vi "NK11003_ONOFF.vi"(8 "error in":errorcluster caption="错误输入（无错误）", 10 "启停":enum16{"启动", "停止"}(ring), 11 "MyIndex":u8) -> (0 "error out":errorcluster caption="错误输出", 3 "OK?":bool)   [LabVIEW 2015]
uses:
  <vilib>/Instr/_visa.llb/VISA Configure Serial Port (Instr).vi
panel:
  out "VISA":refnum<visa-resource-name> caption="VISA资源名称输出"
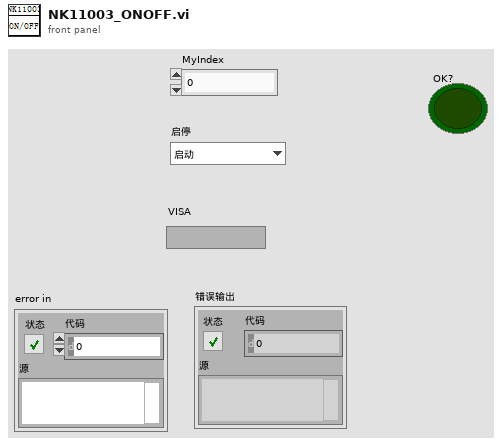
[diagram p1: front panel]
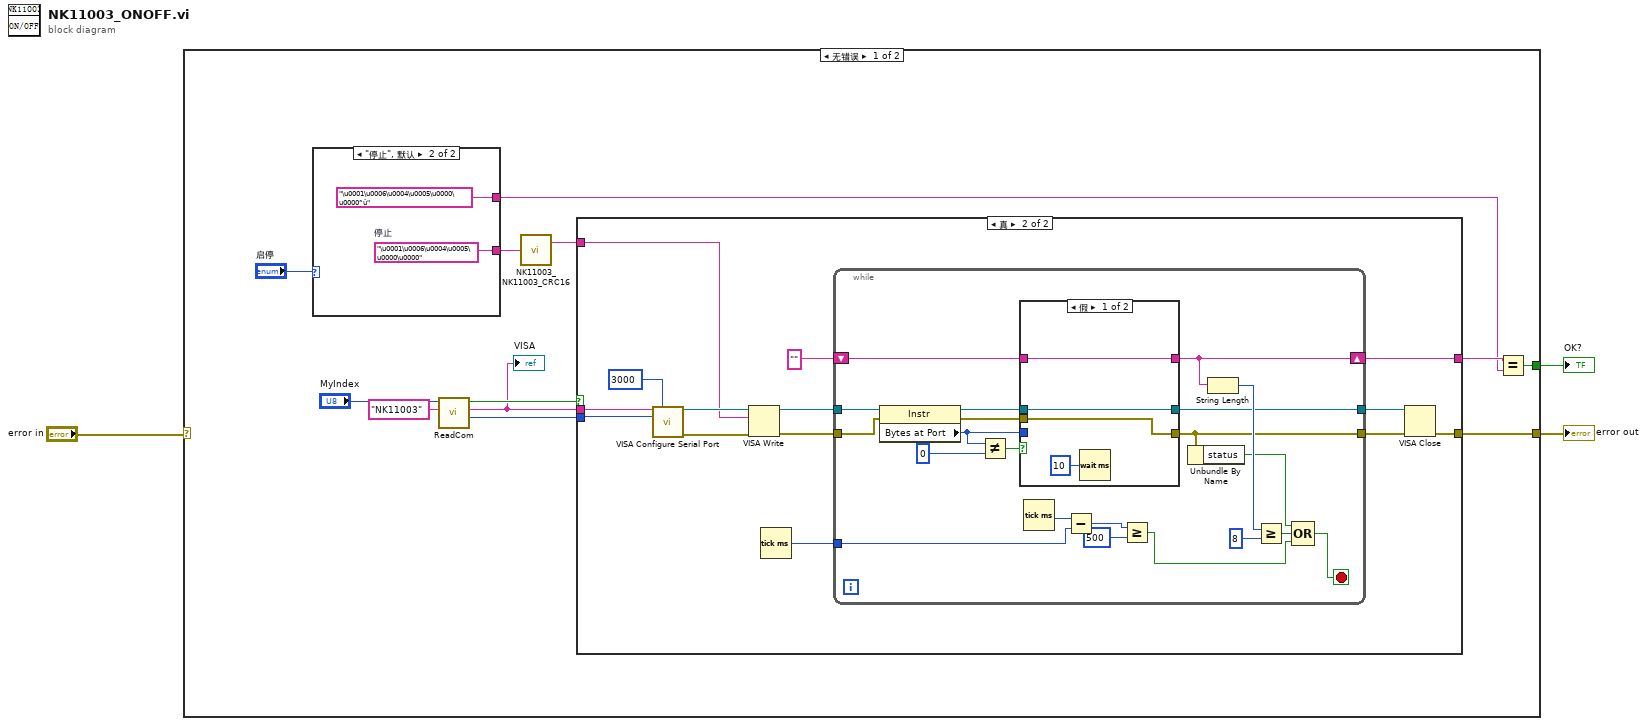
[diagram p0: block diagram]
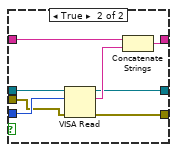
[diagram p3: hidden frame]
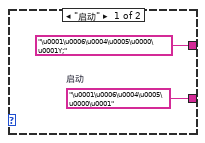
[diagram p4: hidden frame]
diagram:
  n1 = case shown="无错误" "error in" {
    selector: "error in" -> [_ w67]
    tunnel: [w10 _] -> w3
    tunnel: [w4 w67] -> w1
    frame No Error {
      n2 = case shown="\"停止\", 默认" "启停" {
        tunnel: [w64 w66] -> w15
        tunnel: ["\u0001\u0006\u0004\u0005\u0000\u0001Y;" "\u0001\u0006\u0004\u0005\u0000\u0000˜û"] -> w11
        frame "启动" {
          w64 = "\u0001\u0006\u0004\u0005\u0000\u0001"  # 启动
        }
        frame "停止", Default {
          w66 = "\u0001\u0006\u0004\u0005\u0000\u0000"  # 停止
        }
      }
      n3 = call "ReadCom.vi"("仪器名称"="NK11003", "MyIndex"="MyIndex") -> ("Baudrate"=w6:i32, "COM"=w5:string, "OK?"=w7:bool)  [unwired: 7 in]
      "VISA" <- w5
      n4 = call "NK11003_NK11003_CRC16.vi"("input String"=w15) -> ("InPut +CRC"=w13:string)  [unwired: 1 out]
      n5 = case shown="真" w7 {
        tunnel: w13 -> [_ w23]
        tunnel: [_ w22] -> w12
        tunnel: w5 -> [_ w19]
        tunnel: w6 -> [_ w17]
        tunnel: [_ w16] -> w4
        frame False {
        }
        frame True {
          n6 = call-poly "VISA Configure Serial Port"("VISA resource name"=w19, "timeout (10sec)"=u32 3000, "baud rate (9600)"=w17) -> ("VISA resource name out"=w29:refnum<visa-resource-name>, "error out"=w28:errorcluster)  [unwired: 11 in]
          n7 = VISA Write(VISA resource name=w29, write buffer=w23, error in (no error)=w28) -> (VISA resource name out=w26:refnum<visa-resource-name>, error out=w27:errorcluster)  [unwired: 1 out]
          n8 = Tick Count (ms)() -> (millisecond timer value=w24:u32)
          n9 = while {
            tunnel: w27 -> [w30]
            tunnel: w26 -> [w50]
            shift-right: [w43] -> w22
            shift-left: "" -> [w44]
            tunnel: w24 -> [w36]
            tunnel: [w32] -> w21
            tunnel: [w31] -> w20
            stop <- w39 stop-if-true
            n10 = property class="Instr"(reference=w50, error in=w30) -> (reference out=w47:refnum<visa-resource-name>, error out=w45:errorcluster, "Bytes at Port"=w46:u32)
            n11 = Not Equal?(x=w46, y=u32 0) -> (x != y?=w48:bool)
            n12 = case shown="假" w48 {
              tunnel: w47 -> [w51 w62]
              tunnel: w46 -> [_ w61]
              tunnel: w45 -> [w52 w60]
              tunnel: w44 -> [w53 w59]
              tunnel: [w53 w57] -> w43
              tunnel: [w52 w56] -> w31
              tunnel: [w51 w55] -> w32
              frame False {
                n13 = Wait (ms)(milliseconds to wait=u32 10 ("等待时间（毫秒）")) -> ()  [unwired: 1 out]
              }
              frame True {
                n14 = VISA Read(VISA resource name=w62, byte count=w61, error in (no error)=w60) -> (VISA resource name out=w55:refnum<visa-resource-name>, read buffer=w58:string, error out=w56:errorcluster)  [unwired: 1 out]
                n15 = Concatenate Strings(w59, w58) -> (w57:string)
              }
            }
            n16 = Tick Count (ms)() -> (millisecond timer value=w37:u32)
            n17 = Subtract(x=w37, y=w36) -> (x-y=w35:u32)
            n18 = Greater Or Equal?(x=w35, y=u32 500) -> (x >= y?=w33:bool)
            n19 = Unbundle By Name(w31) -> ("status"=w38:bool)
            n20 = String Length(string=w43) -> (length=w42:i32)
            n21 = Greater Or Equal?(x=w42, y=8) -> (x >= y?=w41:bool)
            n22 = Compound Arithmetic op=OR ("复合运算")(w38, w41, w33) -> (w39:bool)
          }
          n23 = VISA Close(VISA resource name=w21, error in (no error)=w20) -> (error out=w16:errorcluster)
        }
      }
      n24 = Equal?(x=w12, y=w11) -> (x = y?=w10:bool)
    }
    frame Error {
    }
  }
  "OK?" <- w3
  "error out" <- w1
